vi "DEMO（队列）.vi"() -> ()   [LabVIEW 2011]
panel:
  out "Output":string
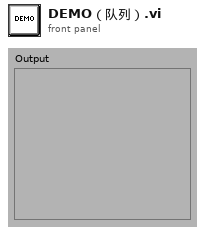
[diagram p1: front panel]
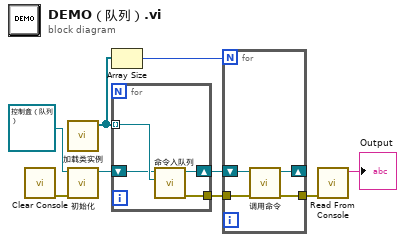
[diagram p0: block diagram]
diagram:
  n1 = call "Clear Console.vi"() -> ("error out"=w2:errorcluster)  [unwired: 11 in]
  n2 = call "加载类实例.vi"() -> ("数组"=w8:refnum<class "命令类.lvclass">[])  [unwired: 10 in, 1 out]
  n3 = call "初始化.vi"("error in (no error)"=w2, "控制盒（队列） 输入"=refnum<class "控制盒（队列）.lvclass"> refnum) -> ("控制盒（队列） 输出"=w9:refnum<class "控制盒（队列）.lvclass">)  [unwired: 8 in, 1 out]
  n4 = Array Size(array=w8) -> (size(s)=w7:i32)
  n5 = for {
    tunnel: w8 -> [w13] mode=indexing
    shift-right: [w11] -> w6
    shift-left: w9 -> [w12]
    tunnel: [w10] -> w4
    n6 = call "命令入队列.vi"("命令类.lvclass"=w13, "控制盒（队列） 输入"=w12) -> ("error out"=w10:errorcluster, "控制盒（队列） 输出"=w11:refnum<class "控制盒（队列）.lvclass">)  [unwired: 8 in]
  }
  n7 = for {
    N: w7 -> [_]
    shift-right: [w16] -> _
    shift-left: w6 -> [w17]
    tunnel: [w15] -> w5
    tunnel: w4 -> [w14]
    n8 = call "调用命令.vi"("error in (no error)"=w14, "控制盒（队列） 输入"=w17) -> ("error out"=w15:errorcluster, "控制盒（队列） 输出"=w16:refnum<class "控制盒（队列）.lvclass">)  [unwired: 8 in]
  }
  n9 = call "Read From Console.vi"("error in (no error)"=w5) -> ("Output"=→"Output":string)  [unwired: 9 in, 1 out]
